vi "3D-Chart Collect.vi"(9 "dATA":cluster{"Barcode":string, "Start time":string}, 10 "Limit":string[](array[string]), 11 "Result":string[](array[string])) -> (0 "File Data":string[](array[string]), 3 "SubItem":string[](array[string]))   [LabVIEW 2011]
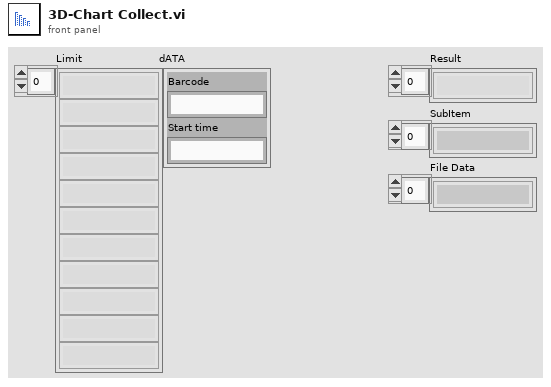
[diagram p1: front panel]
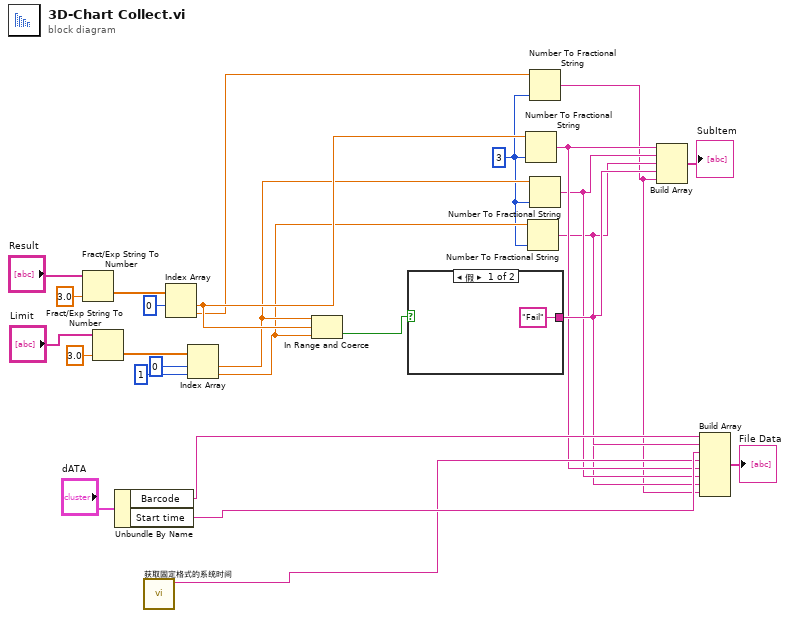
[diagram p0: block diagram]
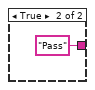
[diagram p2: hidden frame]
diagram:
  w12 = i16 3 ("精度(6)")
  n1 = Fract/Exp String To Number(string="Result", default (0 dbl)=3.0 ("默认(0 DBL)")) -> (number=w19:dbl[])  [unwired: 2 in, 1 out]
  n2 = Fract/Exp String To Number(string="Limit", default (0 dbl)=3.0 ("默认(0 DBL)")) -> (number=w22:dbl[])  [unwired: 2 in, 1 out]
  n3 = Unbundle By Name("dATA") -> ("Barcode"=w9:string, "Start time"=w7:string)
  n4 = call "获取固定格式的系统时间.vi"() -> ("日期/时间字符串"=w6:string)  [unwired: 10 in, 1 out]
  n5 = Index Array(array=w19, index #1=0 ("索引")) -> (element #1=w16:dbl, element #2=w11:dbl)  [unwired: 1 in]
  n6 = Index Array(array=w22, index #1=0 ("索引"), index #2=1 ("索引")) -> (element #1=w15:dbl, element #2=w14:dbl)
  n7 = In Range and Coerce(upper limit=w15, x=w16, lower limit=w14) -> (In Range?=w17:bool)  [unwired: 1 out]
  n8 = case shown="假" w17 {
    tunnel: ["Fail" "Pass"] -> w8
    frame False {
    }
    frame True {
    }
  }
  n9 = Number To Fractional String(number=w16, precision (6)=w12) -> (F-format string=w5:string)  [unwired: 2 in]
  n10 = Number To Fractional String(number=w14, precision (6)=w12) -> (F-format string=w3:string)  [unwired: 2 in]
  n11 = Number To Fractional String(number=w11, precision (6)=w12) -> (F-format string=w2:string)  [unwired: 2 in]
  n12 = Number To Fractional String(number=w15, precision (6)=w12) -> (F-format string=w4:string)  [unwired: 2 in]
  n13 = Build Array(w5, w4, w3, w8, w2) -> (→"SubItem":string[])
  n14 = Build Array(w9, w8, w7, w6, w5, w4, w3, w2) -> (→"File Data":string[])
